vi "getExceptionMessage.vi"(9 "exception":i32, 11 "Job.BuildSpec":refnum<class "Job.BuildSpec.lvclass">) -> (0 "exception message":string, 1 "exception dup":i32, 3 "warning?":bool)   [LabVIEW 2013, in "Job.BuildSpec.lvclass"]
uses:
  Job.BuildSpec.lvclass
  <vilib>/LabVIEW Open Source Project/Cron Scheduler/Job/Job.lvclass
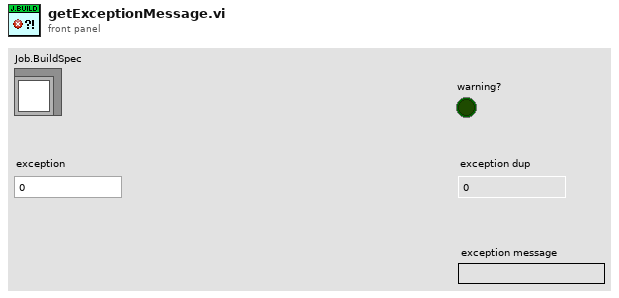
[diagram p1: front panel]
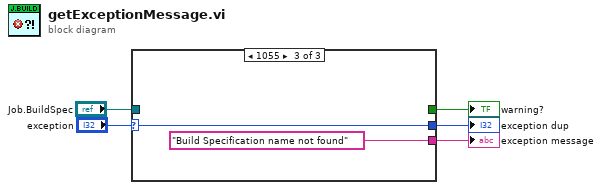
[diagram p0: block diagram]
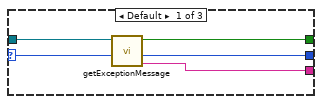
[diagram p2: hidden frame]
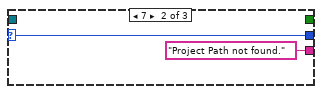
[diagram p3: hidden frame]
diagram:
  n1 = case shown="1055" "exception" {
    selector: "exception" -> [w6 w12 w14]
    tunnel: [w10 "Project Path not found." ("exception message") "Build Specification name not found" ("exception message")] -> w5
    tunnel: [w9 w12 w14] -> w4
    tunnel: [w8 _ _] -> w3
    tunnel: "Job.BuildSpec" -> [w7 _ _]
    frame Default {
      n2 = call-parent "getExceptionMessage.vi"("exception"=w6, "Job in"=w7) -> ("exception message"=w10:string, "exception dup"=w9:i32, "warning?"=w8:bool)  [unwired: 7 in]
    }
    frame 7 {
    }
    frame 1055 {
    }
  }
  "exception dup" <- w4
  "exception message" <- w5
  "warning?" <- w3
